vi "Parameter Setup(Functional).vi"() -> (2 "Channel(s) (out)":u16(ring) items=["1+2", "1", "2", "3"], 3 "Number of Units(out)":i32 min=1 max=32 step=1)   [LabVIEW 2024]
panel:
  in  "Channel(s)":u16(ring) items=["1+2", "1", "2", "3"]
  in  "Enter":bool
  in  "Number of Units":i32=1 min=1 max=32 step=1
  # "Please Enter Number of Units"
  # "Legend:\nChannel(s): Channels used on\nFrequency Counter (1+2 = 16 and 16)"
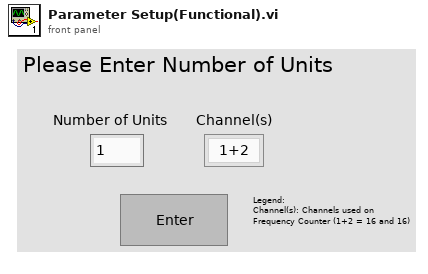
[diagram p1: front panel]
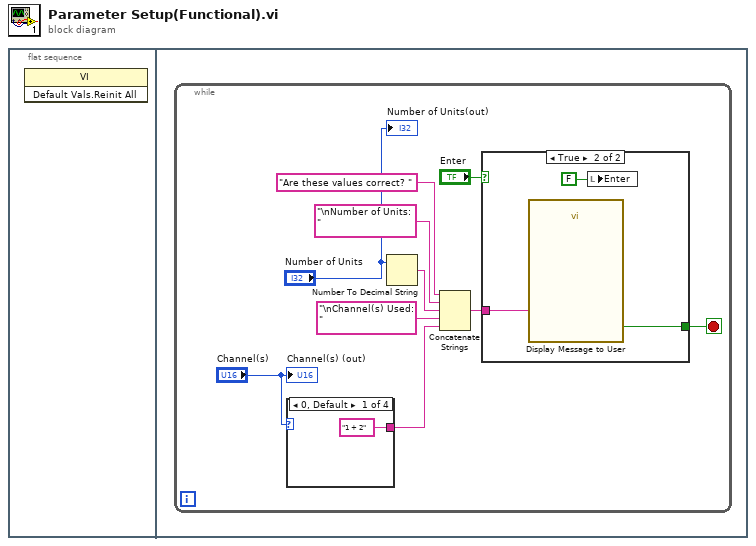
[diagram p0: block diagram]
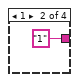
[diagram p2: hidden frame]
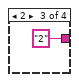
[diagram p3: hidden frame]
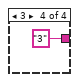
[diagram p4: hidden frame]
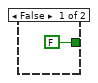
[diagram p5: hidden frame]
diagram:
  n1 = flat-sequence {
    frame #0 {
      n2 = invoke class="VI" method="Default Vals.Reinit All"() -> ()  [unwired: 3 in, 3 out]
    }
    frame #1 {
      n3 = while {
        stop <- w9 stop-if-true
        n4 = case shown="0, Default" "Channel(s)" {
          tunnel: ["1 + 2" "1" "2" "3"] -> w1
          frame 0, Default {
          }
          frame 1 {
          }
          frame 2 {
          }
          frame 3 {
          }
        }
        n5 = Number To Decimal String(number="Number of Units") -> (decimal integer string=w4:string)  [unwired: 1 in]
        n6 = Concatenate Strings("Are these values correct? ", "\nNumber of Units: " ("string"), w4, "\nChannel(s) Used: " ("string"), w1) -> (w6:string)
        n7 = case shown="True" "Enter" {
          tunnel: [FALSE w17] -> w9
          tunnel: w6 -> [_ w16]
          frame False {
          }
          frame True {
            n8 = call "Display Message to User"("Message"=w16) -> ("Yes"=w17:bool)  [unwired: 9 in, 1 out]
            n9 = local write "Enter"(FALSE ("Enter")) -> ()
          }
        }
        "Number of Units(out)" <- "Number of Units"
        "Channel(s) (out)" <- "Channel(s)"
      }
    }
  }
